vi "_IFBOX_CNT.vi"(6 "6501Dev#":i16=1, 7 "IFBOX":T1={" Output"=2, "YIG Fc(GHz)"=8.0, " Filter"=3, "Input"=2} {"Input" items=["1:Pol 0"=1, "2:Pol 1"=2, "3:dummy"=3, "4:NoiseSource"=4]; "Filter" items=["1:YIG"=1, "2:direct"=2, "3:4-12BPF"=3, "4:direct 4-12BPF"=4]; "Output" items=["1:Speana"=1, "2:PowerMeter"=2, "3:dummy"=3, "4:TPD"=4]}) -> ()   [LabVIEW 2017]
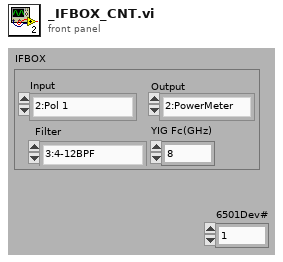
[diagram p1: front panel]
types:
  T1 = cluster{" Output":u16, "YIG Fc(GHz)":dbl, " Filter":u16, "Input":u16}
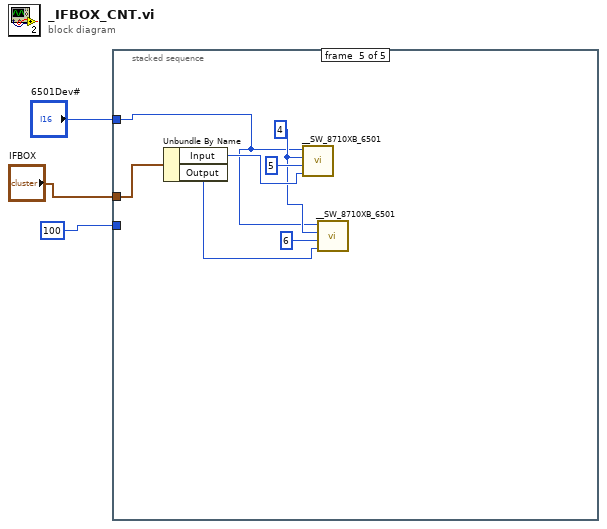
[diagram p0: block diagram]
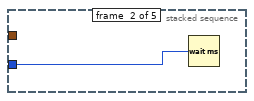
[diagram p3: hidden frame]
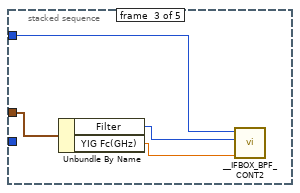
[diagram p4: hidden frame]
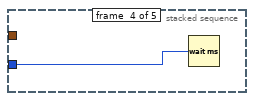
[diagram p5: hidden frame]
diagram:
  n1 = stacked-sequence {
    tunnel: "IFBOX" -> [_ _ w8 _ w16]
    tunnel: 100 -> [_ w4 _ w9 _]
    tunnel: "6501Dev#" -> [_ _ w5 _ w10]
    frame #0 {
    }
    frame #1 {
      n2 = Wait (ms)(milliseconds to wait=w4) -> ()  [unwired: 1 out]
    }
    frame #2 {
      n3 = Unbundle By Name(w8) -> ("Filter"=w6:u16, "YIG Fc(GHz)"=w7:dbl)
      n4 = call "__IFBOX_BPF_CONT2.vi"("YIG frq(GHz) 2"=w7, "フィルター（1:YIG,2:direct,3:4-12BPF,4:direct4-12BPF）"=w6, "Dev#"=w5) -> ()  [unwired: 1 in]
    }
    frame #3 {
      n5 = Wait (ms)(milliseconds to wait=w9) -> ()  [unwired: 1 out]
    }
    frame #4 {
      w11 = 4
      n6 = Unbundle By Name(w16) -> ("Input"=w15:u16, "Output"=w12:u16)
      n7 = call "__SW_8710XB_6501.vi"("Path(1..6)"=w15, "ch(1..6)"=5, "bit(4or6)"=w11, "Dev(1,2..)"=w10) -> ()
      n8 = call "__SW_8710XB_6501.vi"("Path(1..6)"=w12, "ch(1..6)"=6, "bit(4or6)"=w11, "Dev(1,2..)"=w10) -> ()
    }
  }
